vi "Read Color of jedi sword.vi"(8 "error in (no error)":errorcluster, 11 "Jedi in":refnum<class "Jedi.lvclass">) -> (0 "error out":errorcluster, 2 "Color of jedi sword":u32(colorbox), 3 "Jedi out":refnum<class "Jedi.lvclass">)   [LabVIEW 2021, in "Jedi.lvclass"]
uses:
  Jedi.lvclass
  Jedi.lvclass/Jedi.ctl
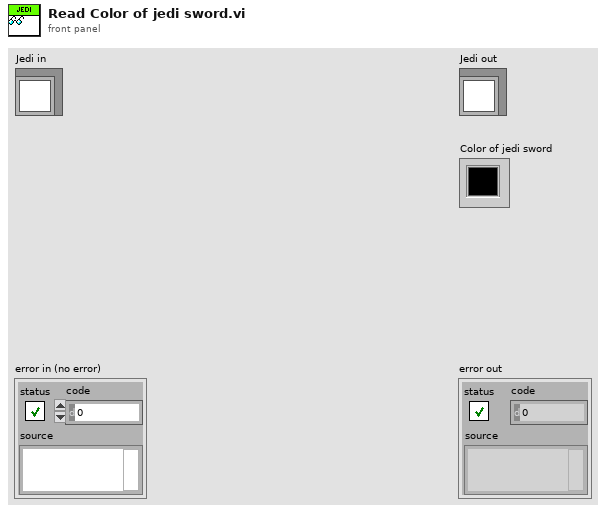
[diagram p1: front panel]
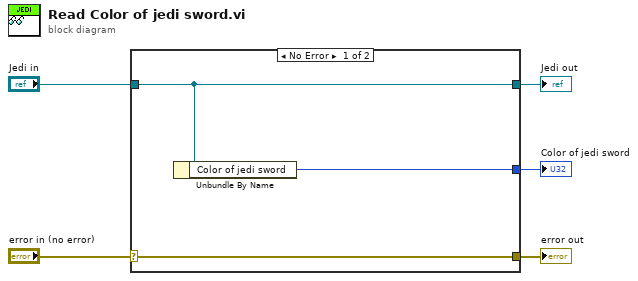
[diagram p0: block diagram]
diagram:
  n1 = case shown="No Error" "error in (no error)" {
    selector: "error in (no error)" -> [w8 w9]
    tunnel: [w8 w9] -> w4
    tunnel: [w7 w10] -> w2
    tunnel: "Jedi in" -> [w7 w10]
    tunnel: [w6 _] -> w1
    frame No Error {
      n2 = Unbundle By Name(w7) -> ("Color of jedi sword"=w6:u32)
    }
    frame Error {
    }
  }
  "error out" <- w4
  "Jedi out" <- w2
  "Color of jedi sword" <- w1
